vi "Save File.vi"(7 "error codes file":path, 8 "error in (no error)":errorcluster, 9 "errors":T1[](array[typedef]), 10 "comment":string, 11 "family":T2) -> (0 "error out":errorcluster)   [LabVIEW 2017, in "Error File Management.lvlib"]
uses:
  Error File Management.lvlib
  Controls/NI Family.ctl
  Controls/NI Error.ctl
  <vilib>/xml/Load XML File.vi
  <vilib>/xml/Close Reference(Node).vi
  <vilib>/xml/NI_XML.lvlib
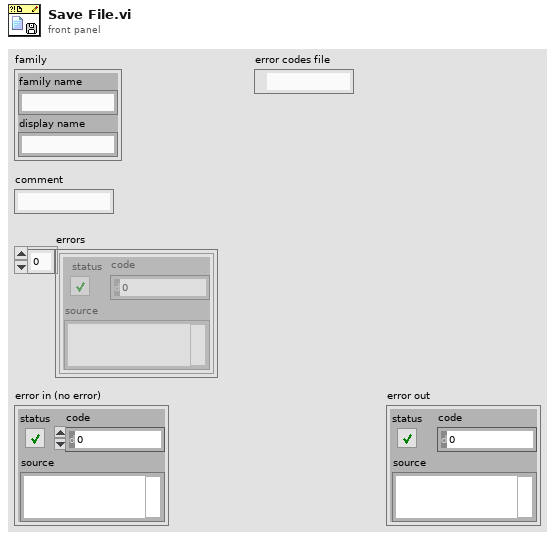
[diagram p1: front panel]
types:
  T1 = typedef "Error File Management.lvlib/NI Error.ctl" = errorcluster
  T2 = typedef "Error File Management.lvlib/NI Family.ctl" = cluster{"family name":string, "display name":string}
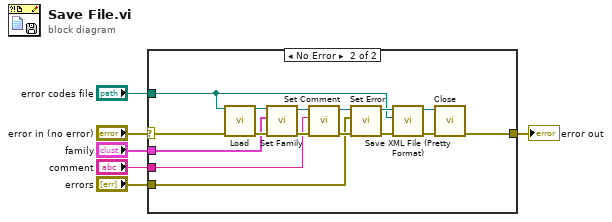
[diagram p0: block diagram]
diagram:
  n1 = case shown="No Error" "error in (no error)" {
    selector: "error in (no error)" -> [w7 w8]
    tunnel: "family" -> [_ w21]
    tunnel: "comment" -> [_ w20]
    tunnel: "errors" -> [_ w11]
    tunnel: "error codes file" -> [_ w10]
    tunnel: [w7 w9] -> w1
    frame Error {
    }
    frame No Error {
      n2 = call-poly <vilib>:"Load.vi"("path to XML document"=w10, "error in (no error)"=w8) -> ("DOM document out"=w13:refnum<k20>, "error out"=w23:errorcluster)  [unwired: 11 in, 1 out]
      n3 = call "Set Family.vi"("error in (no error)"=w23, "family"=w21, "DOM document in"=w13) -> ("error out"=w22:errorcluster, "DOM document out"=w12:refnum<k20>)  [unwired: 7 in]
      n4 = call "Set Comment.vi"("error in (no error)"=w22, "comment"=w20, "DOM document in"=w12) -> ("error out"=w16:errorcluster, "DOM document out"=w17:refnum<k20>)  [unwired: 7 in]
      n5 = call "Set Error.vi"("error in (no error)"=w16, "errors"=w11, "DOM document in"=w17) -> ("error out"=w15:errorcluster, "DOM document out"=w14:refnum<k20>)  [unwired: 7 in]
      n6 = call "Save XML File (Pretty Format).vi"("error in (no error)"=w15, "XML file path"=w10, "DOM document in"=w14) -> ("error out"=w19:errorcluster, "DOM document out"=w18:refnum<k20>)  [unwired: 6 in, 1 out]
      n7 = call-poly <vilib>:"Close.vi"("error in (no error)"=w19, "node"=w18) -> ("error out"=w9:errorcluster)  [unwired: 7 in]
    }
  }
  "error out" <- w1
